vi "UIManager.CreateRequests.vi"(8 "error in (no error)":errorcluster) -> (0 "error out":errorcluster, 3 "Requests":T1)   [LabVIEW 2024, in "UIManager.lvclass"]
uses:
  UIManager.lvclass
  Request Events--cluster.ctl
  Do Something Args.ctl
  JQMHCore/Module/Reply.ctl
  Prepare Args.ctl
  Show Args.ctl
  GetContents Args.ctl
  UIManager.lvclass/UIManager.ctl
  JQMHCore/Module/RQMHModule.lvclass
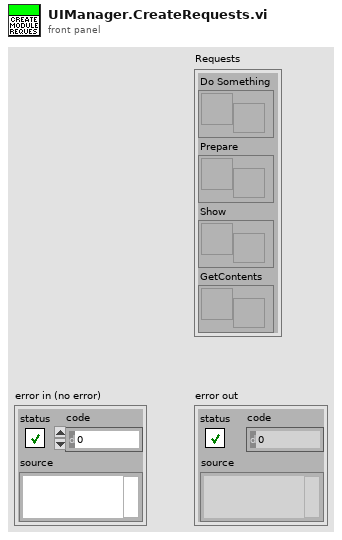
[diagram p1: front panel]
types:
  T1 = typedef "UIManager.lvclass/Request Events--cluster.ctl" = cluster{"Do Something":refnum<user-event>, "Prepare":refnum<user-event>, "Show":refnum<user-event>, "GetContents":refnum<user-event>}
  T2 = typedef "UIManager.lvclass/Prepare Args.ctl" = cluster{"String":string}
  T3 = typedef "RQMHModule.lvclass/Reply.ctl" = cluster{"Expects Reply":bool, "Reply":refnum<notifier>}
  T4 = typedef "UIManager.lvclass/Show Args.ctl" = cluster{"String":string}
  T5 = typedef "UIManager.lvclass/GetContents Args.ctl" = cluster{"String":string}
  T6 = typedef "UIManager.lvclass/Do Something Args.ctl" = cluster{"Msg":string}
  T7 = cluster{"Do Something Args":T6, "Reply Payload":T3}
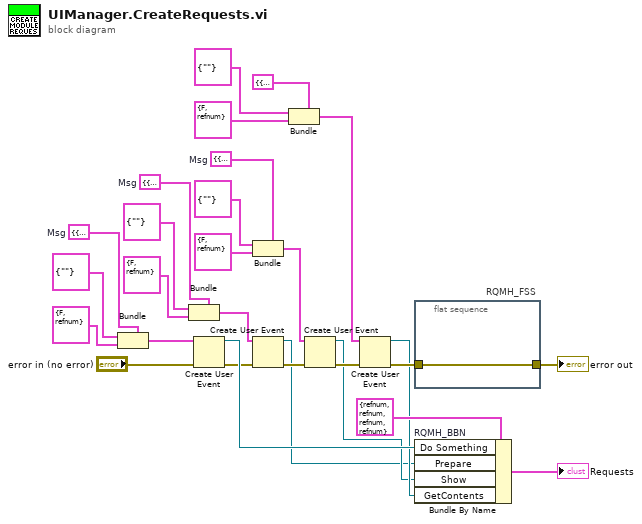
[diagram p0: block diagram]
diagram:
  w3 = cluster{"Prepare Args":T2, "Reply":T3} {"Prepare Args"={"String"=""}, "Reply"={"Expects Reply"=FALSE, "Reply"=refnum}}  # Msg
  w6 = cluster{"Show Args":T4, "Reply":T3} {"Show Args"={"String"=""}, "Reply"={"Expects Reply"=FALSE, "Reply"=refnum}}  # Msg
  w22 = T7 {"Do Something Args"={"Msg"=""}, "Reply Payload"={"Expects Reply"=FALSE, "Reply"=refnum}}  # Msg
  n1 = Bundle(cluster=w22, "Do Something Args"=T6 {"Msg"=""}, "Reply Payload"=T3 {"Expects Reply"=FALSE, "Reply"=refnum}) -> (w25:T7)
  n2 = Bundle(cluster=w3, "Prepare Args"=T2 {"String"=""}, "Reply"=T3 {"Expects Reply"=FALSE, "Reply"=refnum}) -> (w2:cluster{"Prepare Args":T2, "Reply":T3})
  n3 = Create User Event(user event datatype=w25, error in="error in (no error)") -> (user event=w21:refnum<user-event>, error out=w19:errorcluster)
  n4 = Bundle(cluster=w6, "Show Args"=T4 {"String"=""}, "Reply"=T3 {"Expects Reply"=FALSE, "Reply"=refnum}) -> (w9:cluster{"Show Args":T4, "Reply":T3})
  n5 = Create User Event(user event datatype=w2, error in=w19) -> (user event=w1:refnum<user-event>, error out=w18:errorcluster)
  n6 = Bundle(cluster=cluster{"Args":T5, "Reply":T3} {"Args"={"String"=""}, "Reply"={"Expects Reply"=FALSE, "Reply"=refnum}} ("Msg"), "Args"=T5 {"String"=""} ("GetContents Args"), "Reply"=T3 {"Expects Reply"=FALSE, "Reply"=refnum}) -> (w14:cluster{"Args":T5, "Reply":T3})
  n7 = Create User Event(user event datatype=w9, error in=w18) -> (user event=w7:refnum<user-event>, error out=w17:errorcluster)
  n8 = Create User Event(user event datatype=w14, error in=w17) -> (user event=w11:refnum<user-event>, error out=w16:errorcluster)
  n9 = flat-sequence "RQMH_FSS" {
    tunnel: [w29] -> w20
    tunnel: w16 -> [w29]
    frame #0 {
    }
  }
  n10 = Bundle By Name "RQMH_BBN"(cluster=T1 {"Do Something"=refnum, "Prepare"=refnum, "Show"=refnum, "GetContents"=refnum} ("Requests"), "Do Something"=w21, "Prepare"=w1, "Show"=w7, "GetContents"=w11) -> (→"Requests":T1)
  "error out" <- w20
